vi "CurrLim_AmpsToInt.vi"(11 "Current Limit (Amps)":dbl=1.0) -> (3 "Numeric":i16)   [LabVIEW 2011]
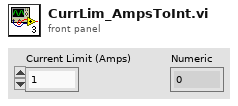
[diagram p1: front panel]
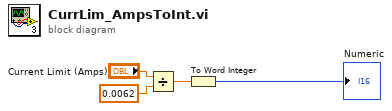
[diagram p0: block diagram]
diagram:
  n1 = Divide(x="Current Limit (Amps)", y=0.0062) -> (x/y=w3:dbl)
  n2 = To Word Integer(number=w3) -> (16bit integer=→"Numeric":i16)
